vi "Set_Frequency.vi"(7 "Menu Ring":u16(ring) items=["Channel 1", "Channel 2"], 9 "Frequency":dbl=100.0, 11 "VISA resource name":refnum<visa-resource-name>="USB0::0x0699::0x0347::C036837::INSTR") -> (3 "VISA resource name out":refnum<visa-resource-name>)   [LabVIEW 2011]
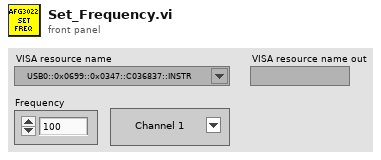
[diagram p1: front panel]
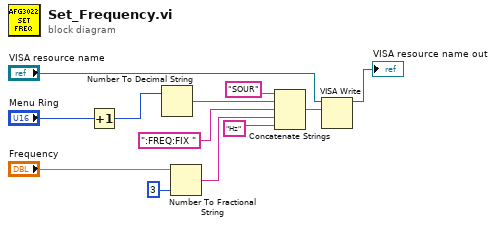
[diagram p0: block diagram]
diagram:
  n1 = Increment(x="Menu Ring") -> (x+1=w5:u16)
  n2 = Number To Decimal String(number=w5) -> (decimal integer string=w4:string)  [unwired: 1 in]
  n3 = Number To Fractional String(number="Frequency", precision (6)=i16 3) -> (F-format string=w9:string)  [unwired: 2 in]
  n4 = Concatenate Strings("SOUR", w4, ":FREQ:FIX " ("string"), w9, "Hz" ("string")) -> (w7:string)
  n5 = VISA Write(VISA resource name="VISA resource name", write buffer=w7) -> (VISA resource name out=→"VISA resource name out":refnum<visa-resource-name>)  [unwired: 1 in, 2 out]
